vi "BiasError.vi"(1 "B":dbl[](array[numeric]), 2 "y":dbl[](array[numeric]), 3 "frequency":dbl) -> (0 "error":dbl)   [LabVIEW 2021]
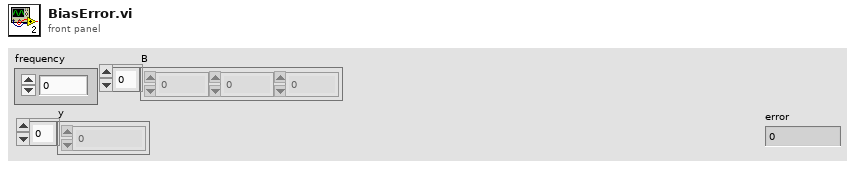
[diagram p1: front panel]
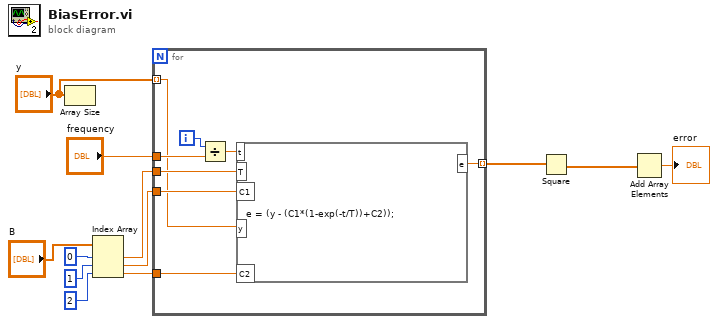
[diagram p0: block diagram]
diagram:
  n1 = Array Size(array="y") -> ()  [unwired: 1 out]
  n2 = Index Array(array="B", index #1=0 ("index"), index #2=1 ("index"), index #3=2 ("index")) -> (element #1=w8:dbl, element #2=w7:dbl, element #3=w6:dbl)
  n3 = for {
    tunnel: [w20] -> w12 mode=indexing
    tunnel: w8 -> [w19]
    tunnel: w7 -> [w18]
    tunnel: w6 -> [w17]
    tunnel: "y" -> [w13] mode=indexing
    tunnel: "frequency" -> [w15]
    i -> [w16]
    n4 = Divide(x=w16, y=w15) -> (x/y=w14:dbl)
    n5 = formula code="e = (y - (C1*(1-exp(-t/T))+C2));"("t"=w14, "T"=w19, "C1"=w18, "C2"=w17, "y"=w13) -> ("e"=w20:dbl)
  }
  n6 = Square(x=w12) -> (x^2=w1:dbl[])
  n7 = Add Array Elements(numeric array=w1) -> (sum=→"error":dbl)
